vi "TC110.vi"(7 "Function":T3=enum."Read command", 8 "Error in":errorcluster, 10 "Settings in":T2) -> (0 "Error out":errorcluster, 1 "Status_string":string, 2 "Settings out":T2, 3 "output cluster":T1)   [LabVIEW 2018]
uses:
  Ctl/Function_of_TC110.ctl
  PublicSubVI/Ctl/_ctl_RT_TurboSettings.ctl
  Example/RS485_TurboPump/Public/Turbopumps/PV Operating adjustment - Cluster.ctl
  Example/RS485_TurboPump/Pfeiffer Vacuum.lvlib
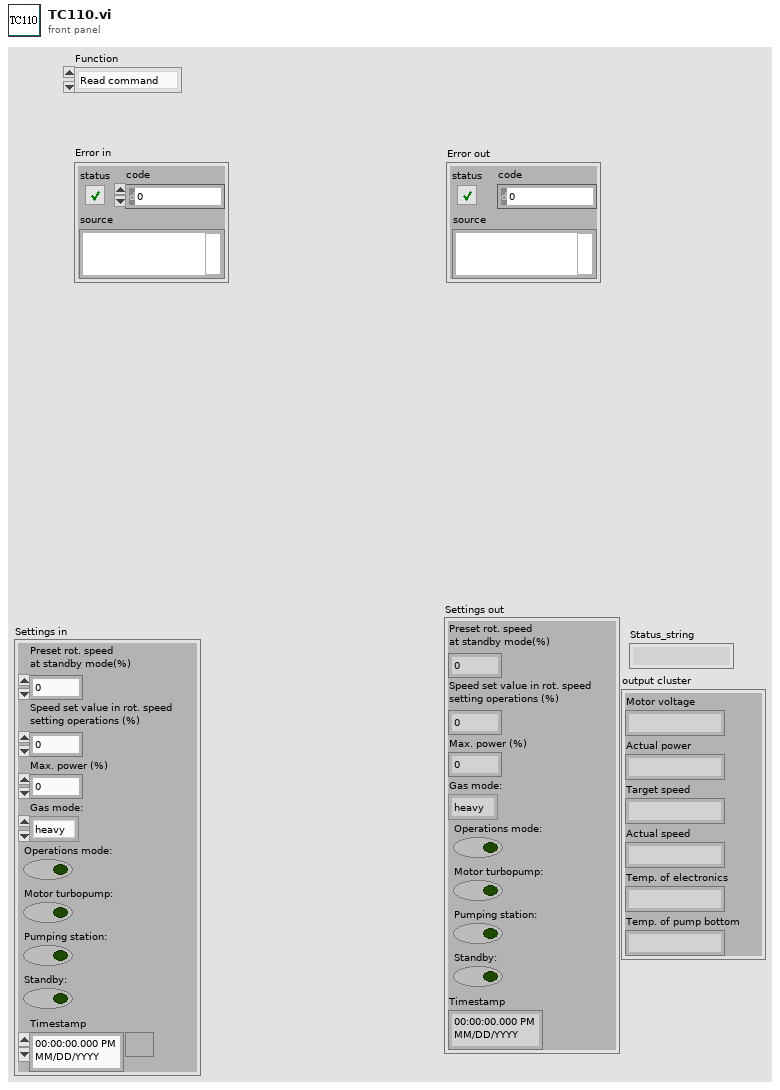
[diagram p1: front panel]
types:
  T1 = cluster{"Motor voltage":string, "Actual power":string, "Target speed":string, "Actual speed":string, "Temp. of electronics":string, "Temp. of pump bottom":string}
  T2 = typedef "_ctl_RT_TurboSettings.ctl" = cluster{"Preset rot. speed \nat standby mode(%)":dbl, "Speed set value in rot. speed \nsetting operations (%)":dbl, "Max. power (%)":dbl, "Gas mode: ":enum16{"heavy", "light", "helium"}, "Operations mode: ":bool, "Motor turbopump: ":bool, "Pumping station: ":bool, "Standby: ":bool, "Timestamp":timestamp}
  T3 = typedef "Function_of_TC110.ctl" = enum16{"Initialisation", "Read status", "Write command", "Read command"}
  T4 = typedef "Pfeiffer Vacuum.lvlib/PV Operating adjustment - Cluster.ctl" = cluster{"Parameter":u16, "Parameter\nread only<->describe":bool, "off<->on":bool, "Rotation speed set value\nin rot. speed setting\noperations [%]":dbl, "Preset rotation Speed\nat Standby mode (%)":dbl, "maximum power\nsetpoint [%]":i32, "Gas mode":u16}
  T5 = enum16{"temperature inverter [°C] (324)", "temperature electronic [°C] (326)", "temperature pump bottom [°C] (330)", "temperature bearing [°C] (342)", "temperature motor [°C] (346)", "temperature rotor [°C] (384)"}
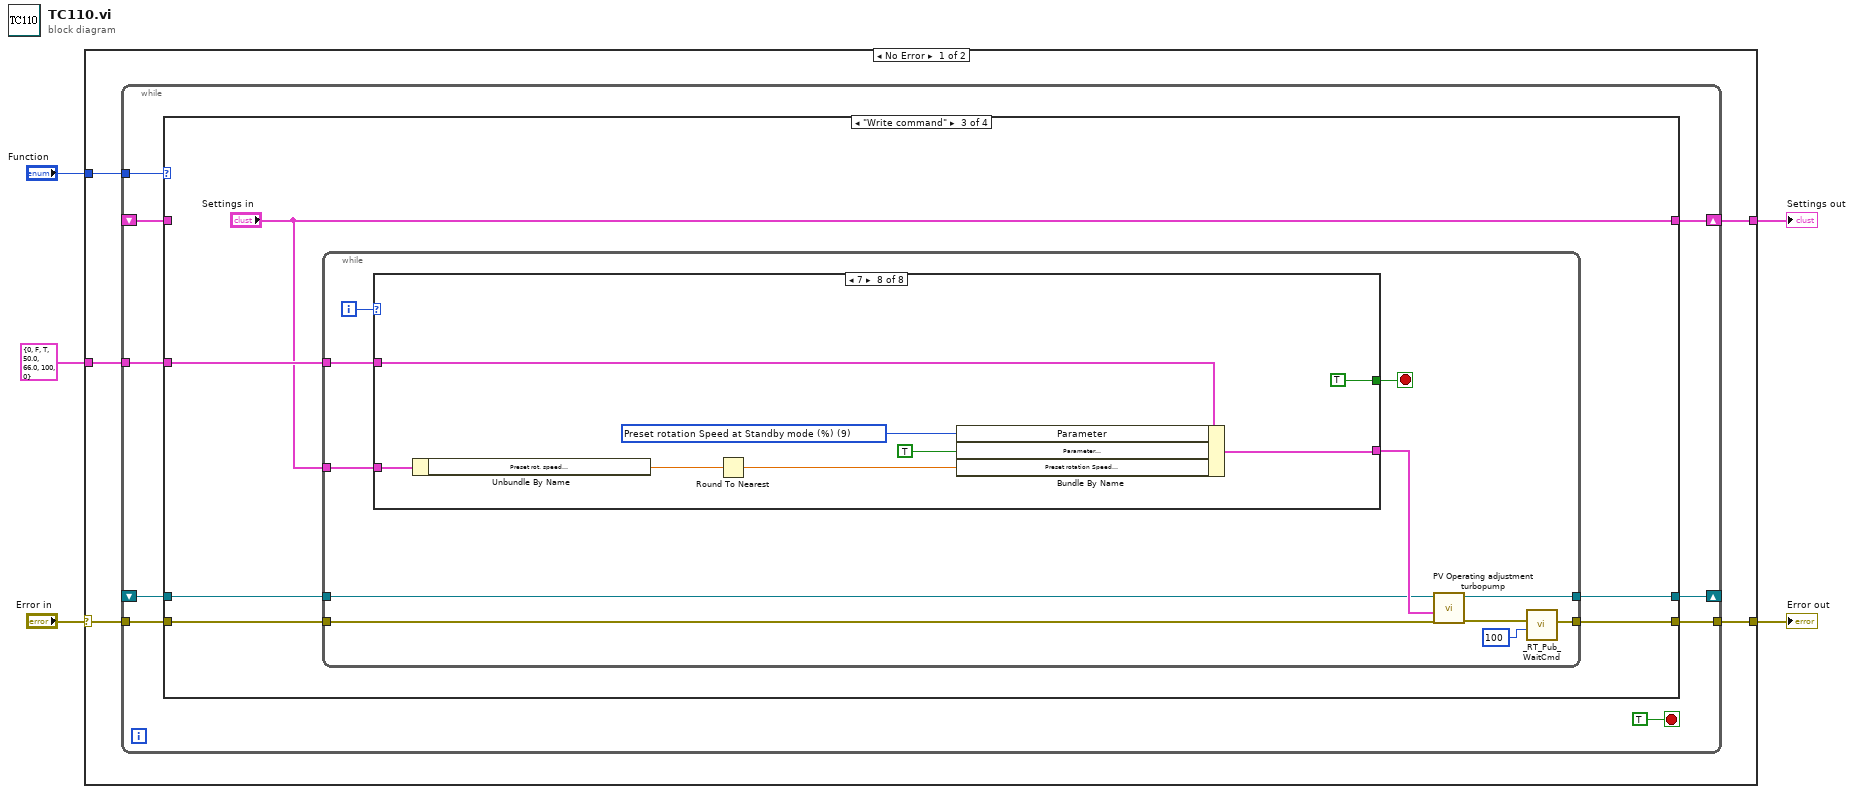
[diagram p0: block diagram]
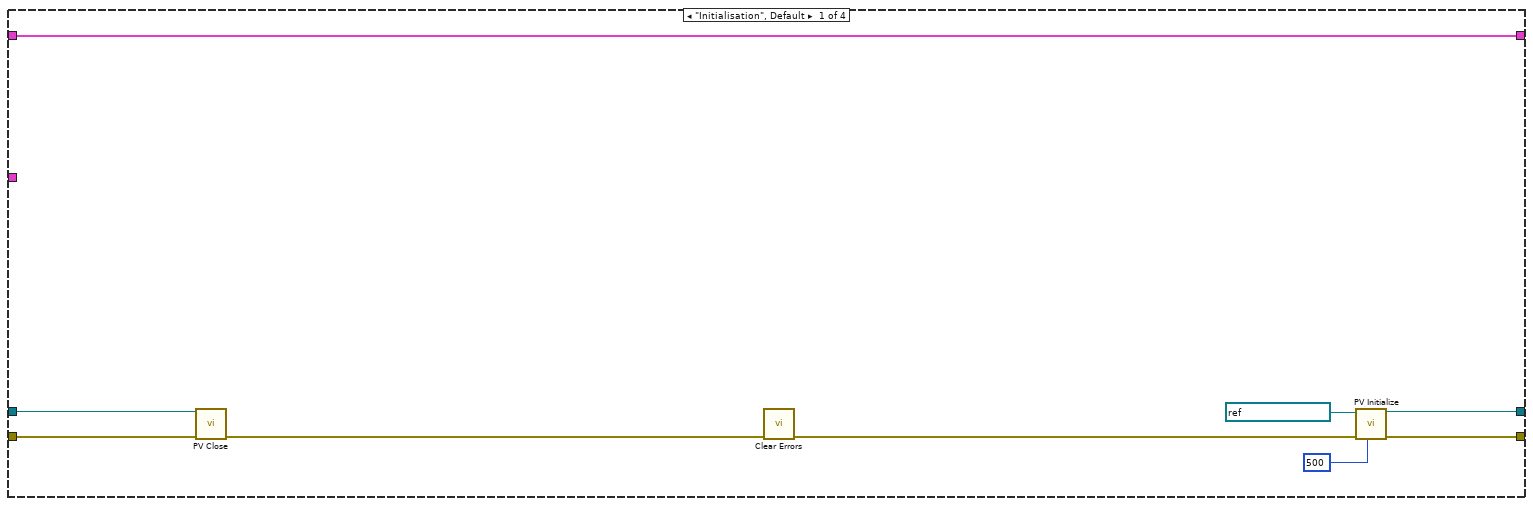
[diagram p2: hidden frame]
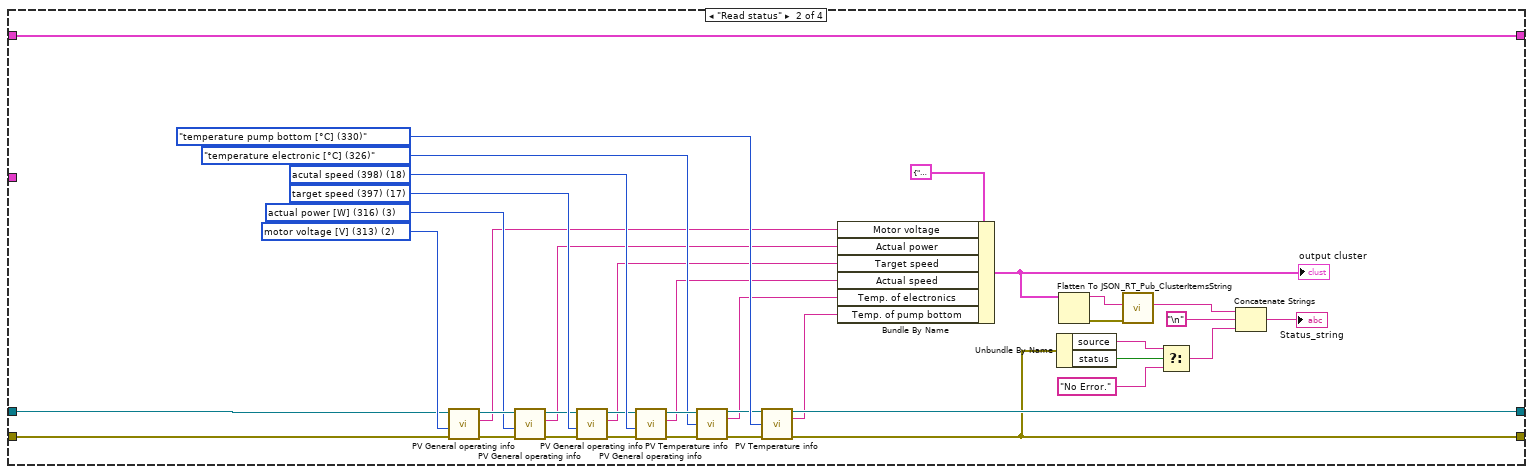
[diagram p3: hidden frame]
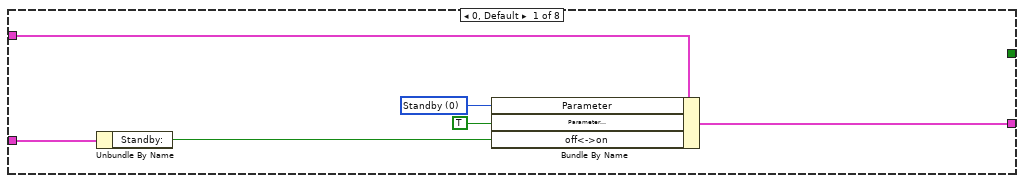
[diagram p4: hidden frame]
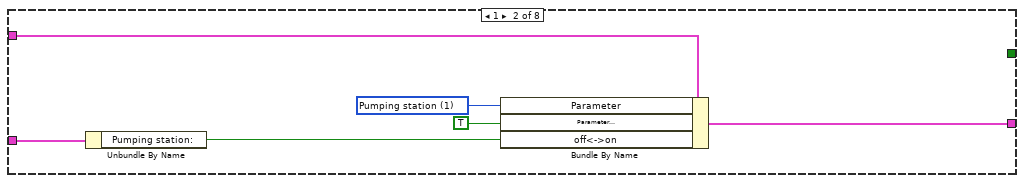
[diagram p5: hidden frame]
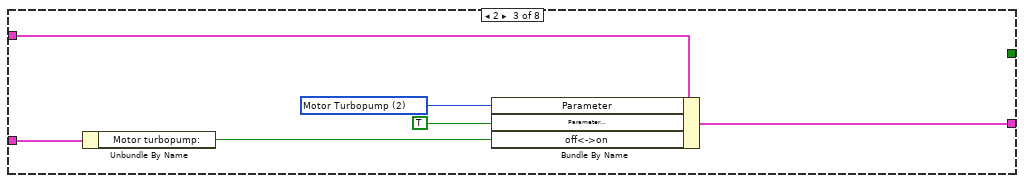
[diagram p6: hidden frame]
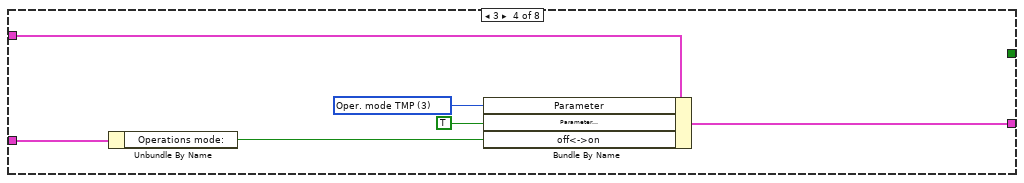
[diagram p7: hidden frame]
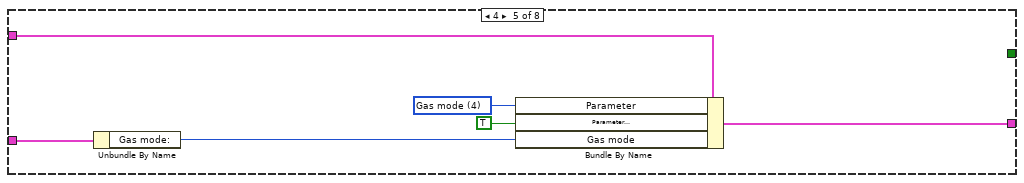
[diagram p8: hidden frame]
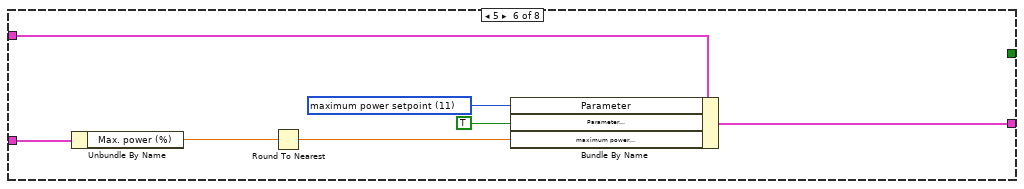
[diagram p9: hidden frame]
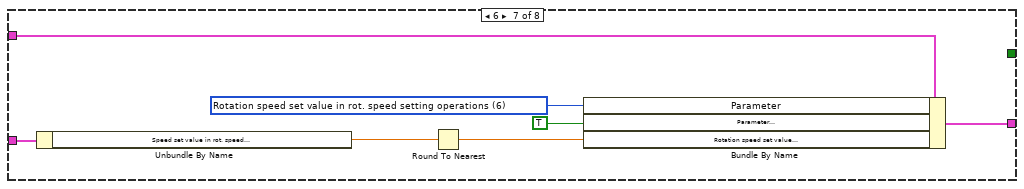
[diagram p10: hidden frame]
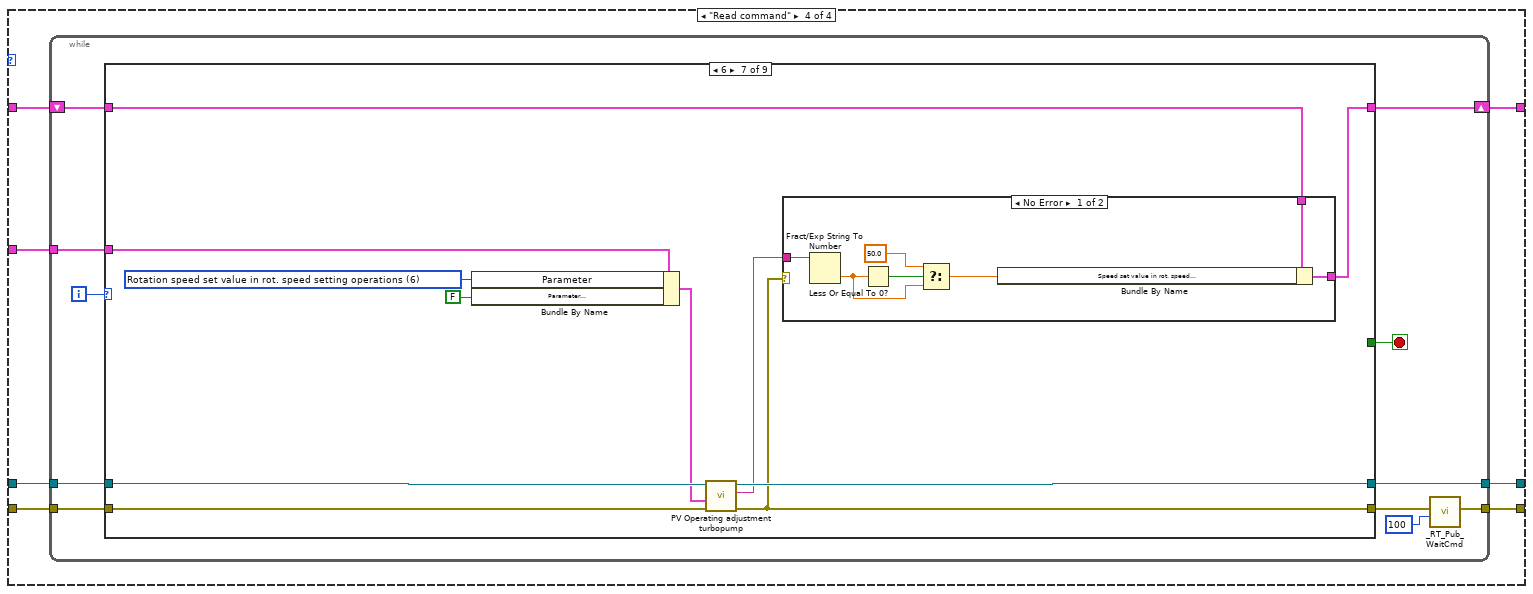
[diagram p11: hidden frame]
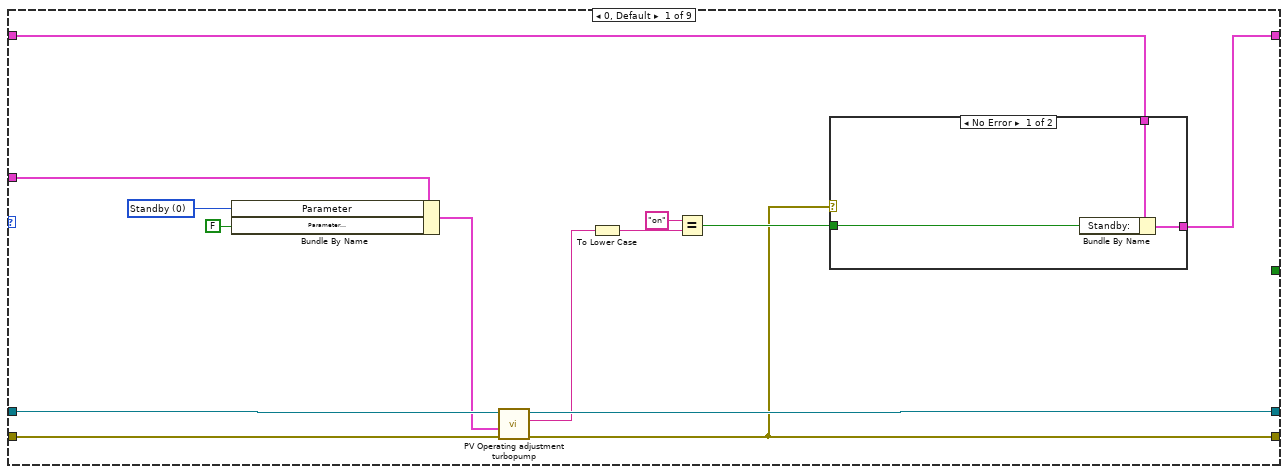
[diagram p12: hidden frame]
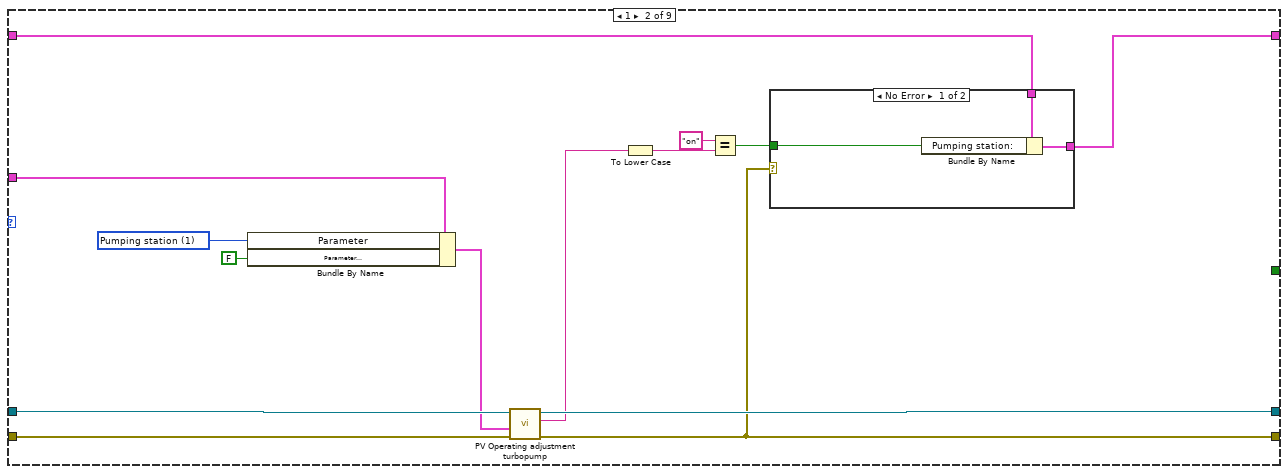
[diagram p14: hidden frame]
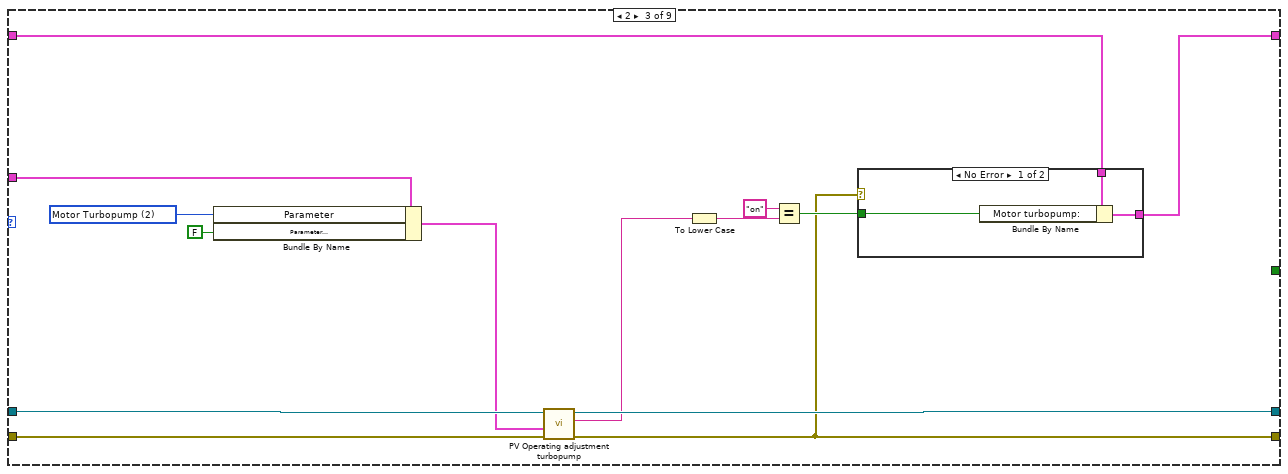
[diagram p16: hidden frame]
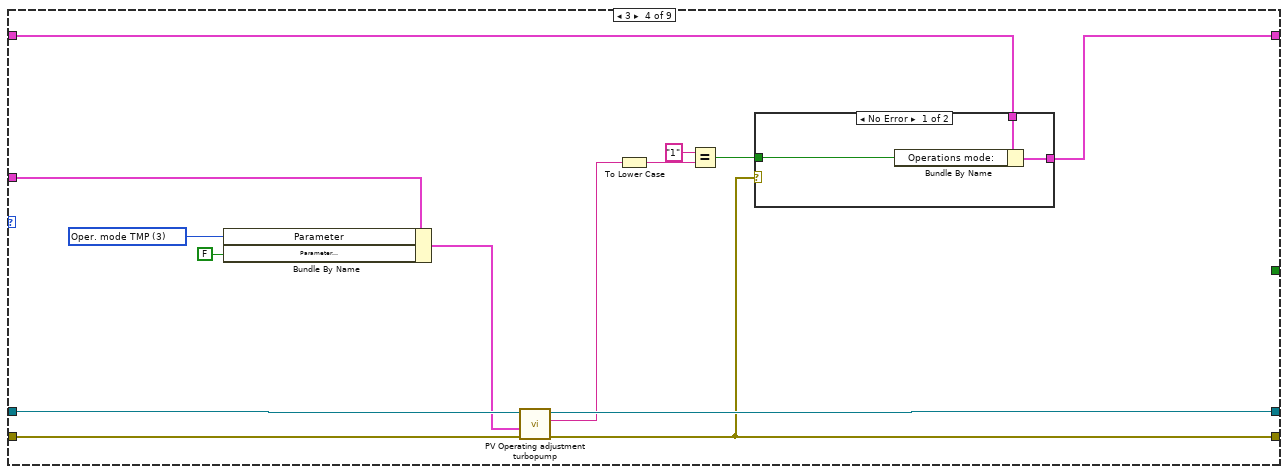
[diagram p18: hidden frame]
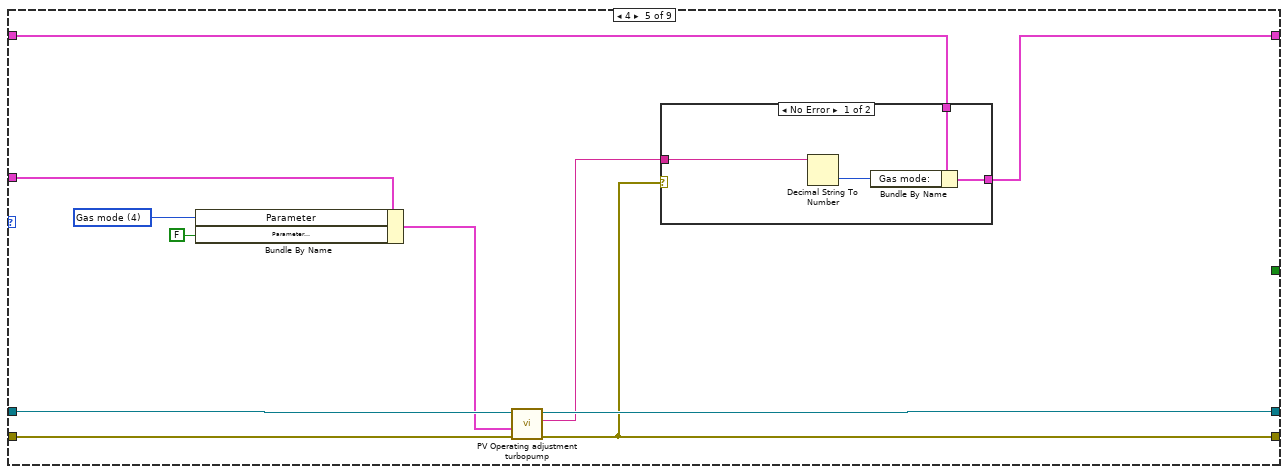
[diagram p20: hidden frame]
diagram:
  n1 = case shown="No Error" "Error in" {
    selector: "Error in" -> [w6 w311]
    tunnel: [w10 w311] -> w5
    tunnel: [w9 _] -> w4
    tunnel: T4 {"Parameter"=0, "Parameter\nread only<->describe"=FALSE, "off<->on"=TRUE, "Rotation speed set value\nin rot. speed setting\noperations [%]"=50.0, "Preset rotation Speed\nat Standby mode (%)"=66.0, "maximum power\nsetpoint [%]"=100, "Gas mode"=0} ("Operating adjustment - Cluster") -> [w8 _]
    tunnel: "Function" -> [w7 _]
    frame No Error {
      n2 = while {
        tunnel: w8 -> [w16]
        tunnel: w7 -> [w14]
        shift-right: [w18] -> w9
        shift-left: _ -> [w15]
        tunnel: w6 -> [w17]
        tunnel: [w19] -> w10
        shift-right: [w13] -> _
        shift-left: _ -> [w11]
        stop <- TRUE stop-if-true
        n3 = case shown="\"Write command\"" w14 {
          tunnel: w17 -> [w24 w30 w70 w140]
          tunnel: [w27 w46 w68 w137] -> w13
          tunnel: w11 -> [w25 w31 w71 w141]
          tunnel: [w26 w39 w69 w138] -> w19
          tunnel: w15 -> [w20 w29 _ w139]
          tunnel: w16 -> [_ _ w72 w142]
          tunnel: [w20 w29 "Settings in" w136] -> w18
          frame "Initialisation", Default {
            n4 = call "PV Close.vi"("VISA session"=w25, "error in (no error)"=w24) -> ("error out"=w23:errorcluster)  [unwired: 13 in]
            n5 = call <vilib>:"Clear Errors.vi"("error in (no error)"=w23) -> ("error out"=w22:errorcluster)  [unwired: 5 in, 1 out]
            n6 = call "PV Initialize.vi"("Timeout Value"=u32 500, "error in (no error)"=w22, "VISA session in"=refnum<visa-resource-name> "ASRL3::INSTR") -> ("error out"=w26:errorcluster, "VISA session out"=w27:refnum<visa-resource-name>)  [unwired: 7 in]
          }
          frame "Read status" {
            w62 = u16 18 items=["nominal speed [Hz] (default) (315)", "intermediate circut current [A] (310)", "motor voltage [V] (313)", "actual power [W] (316)", "operating hours pump [h] (311)", "operating hours drive [h] (314)", "pump cycles (read only) (319)", "status oil sensor (read only) (301)", "speed switchpoint attained (read only) (302)", "overtemperature drive (read only) (304)", "overtemperature pump (read only) (305)", "target speed attained (read only) (306)", "pump accelerates (read only) (307) ", "controlled by remote (300)", "motor phase current [A] (317)", "acceleration / deceleration [rm/s] (336)", "hardware version controller (354)", "target speed (397)", "acutal speed (398)", "nominal speed (399)", "software version control unit (read only) (352)"] ("Parameter")
            w63 = u16 17 items=["nominal speed [Hz] (default) (315)", "intermediate circut current [A] (310)", "motor voltage [V] (313)", "actual power [W] (316)", "operating hours pump [h] (311)", "operating hours drive [h] (314)", "pump cycles (read only) (319)", "status oil sensor (read only) (301)", "speed switchpoint attained (read only) (302)", "overtemperature drive (read only) (304)", "overtemperature pump (read only) (305)", "target speed attained (read only) (306)", "pump accelerates (read only) (307) ", "controlled by remote (300)", "motor phase current [A] (317)", "acceleration / deceleration [rm/s] (336)", "hardware version controller (354)", "target speed (397)", "acutal speed (398)", "nominal speed (399)", "software version control unit (read only) (352)"] ("Parameter")
            w64 = u16 3 items=["nominal speed [Hz] (default) (315)", "intermediate circut current [A] (310)", "motor voltage [V] (313)", "actual power [W] (316)", "operating hours pump [h] (311)", "operating hours drive [h] (314)", "pump cycles (read only) (319)", "status oil sensor (read only) (301)", "speed switchpoint attained (read only) (302)", "overtemperature drive (read only) (304)", "overtemperature pump (read only) (305)", "target speed attained (read only) (306)", "pump accelerates (read only) (307) ", "controlled by remote (300)", "motor phase current [A] (317)", "acceleration / deceleration [rm/s] (336)", "hardware version controller (354)", "target speed (397)", "acutal speed (398)", "nominal speed (399)", "software version control unit (read only) (352)"] ("Parameter")
            w66 = u16 2 items=["nominal speed [Hz] (default) (315)", "intermediate circut current [A] (310)", "motor voltage [V] (313)", "actual power [W] (316)", "operating hours pump [h] (311)", "operating hours drive [h] (314)", "pump cycles (read only) (319)", "status oil sensor (read only) (301)", "speed switchpoint attained (read only) (302)", "overtemperature drive (read only) (304)", "overtemperature pump (read only) (305)", "target speed attained (read only) (306)", "pump accelerates (read only) (307) ", "controlled by remote (300)", "motor phase current [A] (317)", "acceleration / deceleration [rm/s] (336)", "hardware version controller (354)", "target speed (397)", "acutal speed (398)", "nominal speed (399)", "software version control unit (read only) (352)"] ("Parameter")
            n7 = call "PV General operating info.vi"("error in (no error)"=w30, "Parameter"=w66, "VISA session"=w31) -> ("error out"=w59:errorcluster, "response (data)"=w49:string, "dup VISA session"=w65:refnum<visa-resource-name>)  [unwired: 6 in]
            n8 = call "PV General operating info.vi"("error in (no error)"=w59, "Parameter"=w64, "VISA session"=w65) -> ("error out"=w58:errorcluster, "response (data)"=w43:string, "dup VISA session"=w61:refnum<visa-resource-name>)  [unwired: 6 in]
            n9 = call "PV General operating info.vi"("error in (no error)"=w58, "Parameter"=w63, "VISA session"=w61) -> ("error out"=w57:errorcluster, "response (data)"=w44:string, "dup VISA session"=w60:refnum<visa-resource-name>)  [unwired: 6 in]
            n10 = call "PV General operating info.vi"("error in (no error)"=w57, "Parameter"=w62, "VISA session"=w60) -> ("error out"=w53:errorcluster, "response (data)"=w48:string, "dup VISA session"=w56:refnum<visa-resource-name>)  [unwired: 6 in]
            n11 = call "PV Temperature info.vi"("VISA session"=w56, "Parameter"=T5."temperature electronic [°C] (326)", "error in (no error)"=w53) -> ("dup VISA session"=w52:refnum<visa-resource-name>, "response (data)"=w47:string, "error out"=w51:errorcluster)  [unwired: 10 in]
            n12 = call "PV Temperature info.vi"("VISA session"=w52, "Parameter"=T5."temperature pump bottom [°C] (330)", "error in (no error)"=w51) -> ("dup VISA session"=w46:refnum<visa-resource-name>, "response (data)"=w45:string, "error out"=w39:errorcluster)  [unwired: 10 in]
            n13 = Bundle By Name(cluster=T1 {"Motor voltage"="", "Actual power"="", "Target speed"="", "Actual speed"="", "Temp. of electronics"="", "Temp. of pump bottom"=""}, "Motor voltage"=w49, "Actual power"=w43, "Target speed"=w44, "Actual speed"=w48, "Temp. of electronics"=w47, "Temp. of pump bottom"=w45) -> (w42:T1)
            "output cluster" <- w42
            n14 = Unbundle By Name(w39) -> ("source"=w37:string, "status"=w38:bool)
            n15 = Flatten To JSON(anything=w42) -> (JSON string=w41:string, 11:w40:errorcluster)  [unwired: 2 in]
            n16 = call "_RT_Pub_ClusterItemsString.vi"("error in (no error)"=w40, "JSON string"=w41) -> ("result string"=w35:string)  [unwired: 8 in, 1 out]
            n17 = Select(t=w37, s=w38, f="No Error.") -> (s? t:f=w33:string)
            n18 = Concatenate Strings(w35, "\n" ("string"), w33) -> (→"Status_string":string)
          }
          frame "Write command" {
            n19 = while {
              tunnel: "Settings in" -> [w83]
              tunnel: w71 -> [w76]
              tunnel: w70 -> [w75]
              tunnel: [w79] -> w69
              tunnel: w72 -> [w82]
              tunnel: [w73] -> w68
              i -> [w81]
              stop <- w80 stop-if-true
              n20 = case shown="7" w81 {
                tunnel: w83 -> [w87 w93 w99 w105 w111 w118 w125 w133]
                tunnel: w82 -> [w89 w95 w101 w107 w113 w120 w127 w135]
                tunnel: [_ _ _ _ _ _ _ TRUE] -> w80
                tunnel: [w84 w90 w96 w102 w108 w114 w121 w128] -> w77
                frame 0, Default {
                  w85 = u16 0 items=[" Standby", " Pumping station", " Motor Turbopump", " Oper. mode TMP", " Gas mode", " Operating mode drive unit", " Rotation speed set value in rot. speed setting operations", " Set rotation speed TMP [Hz] (read only)", " Actual rotation speed TMP [Hz] (read only)", " Preset rotation Speed at Standby mode (%)", " Max. rotations speed ", " maximum power setpoint"] ("Parameter")
                  n21 = Unbundle By Name(w87) -> ("Standby:"=w86:bool)
                  n22 = Bundle By Name(cluster=w89, "Parameter"=w85, "Parameter\nread only<->describe"=TRUE ("Parameter\nread only<->describe"), "off<->on"=w86) -> (w84:T4)
                }
                frame 1 {
                  w91 = u16 1 items=[" Standby", " Pumping station", " Motor Turbopump", " Oper. mode TMP", " Gas mode", " Operating mode drive unit", " Rotation speed set value in rot. speed setting operations", " Set rotation speed TMP [Hz] (read only)", " Actual rotation speed TMP [Hz] (read only)", " Preset rotation Speed at Standby mode (%)", " Max. rotations speed ", " maximum power setpoint"] ("Parameter")
                  n23 = Unbundle By Name(w93) -> ("Pumping station:"=w92:bool)
                  n24 = Bundle By Name(cluster=w95, "Parameter"=w91, "Parameter\nread only<->describe"=TRUE ("Parameter\nread only<->describe"), "off<->on"=w92) -> (w90:T4)
                }
                frame 2 {
                  w97 = u16 2 items=[" Standby", " Pumping station", " Motor Turbopump", " Oper. mode TMP", " Gas mode", " Operating mode drive unit", " Rotation speed set value in rot. speed setting operations", " Set rotation speed TMP [Hz] (read only)", " Actual rotation speed TMP [Hz] (read only)", " Preset rotation Speed at Standby mode (%)", " Max. rotations speed ", " maximum power setpoint"] ("Parameter")
                  n25 = Unbundle By Name(w99) -> ("Motor turbopump:"=w98:bool)
                  n26 = Bundle By Name(cluster=w101, "Parameter"=w97, "Parameter\nread only<->describe"=TRUE ("Parameter\nread only<->describe"), "off<->on"=w98) -> (w96:T4)
                }
                frame 3 {
                  w103 = u16 3 items=[" Standby", " Pumping station", " Motor Turbopump", " Oper. mode TMP", " Gas mode", " Operating mode drive unit", " Rotation speed set value in rot. speed setting operations", " Set rotation speed TMP [Hz] (read only)", " Actual rotation speed TMP [Hz] (read only)", " Preset rotation Speed at Standby mode (%)", " Max. rotations speed ", " maximum power setpoint"] ("Parameter")
                  n27 = Unbundle By Name(w105) -> ("Operations mode:"=w104:bool)
                  n28 = Bundle By Name(cluster=w107, "Parameter"=w103, "Parameter\nread only<->describe"=TRUE ("Parameter\nread only<->describe"), "off<->on"=w104) -> (w102:T4)
                }
                frame 4 {
                  w109 = u16 4 items=[" Standby", " Pumping station", " Motor Turbopump", " Oper. mode TMP", " Gas mode", " Operating mode drive unit", " Rotation speed set value in rot. speed setting operations", " Set rotation speed TMP [Hz] (read only)", " Actual rotation speed TMP [Hz] (read only)", " Preset rotation Speed at Standby mode (%)", " Max. rotations speed ", " maximum power setpoint"] ("Parameter")
                  n29 = Unbundle By Name(w111) -> ("Gas mode:"=w110:enum16{"heavy", "light", "helium"})
                  n30 = Bundle By Name(cluster=w113, "Parameter"=w109, "Parameter\nread only<->describe"=TRUE ("Parameter\nread only<->describe"), "Gas mode"=w110) -> (w108:T4)
                }
                frame 5 {
                  w116 = u16 11 items=[" Standby", " Pumping station", " Motor Turbopump", " Oper. mode TMP", " Gas mode", " Operating mode drive unit", " Rotation speed set value in rot. speed setting operations", " Set rotation speed TMP [Hz] (read only)", " Actual rotation speed TMP [Hz] (read only)", " Preset rotation Speed at Standby mode (%)", " Max. rotations speed ", " maximum power setpoint"] ("Parameter")
                  n31 = Unbundle By Name(w118) -> ("Max. power (%)"=w117:dbl)
                  n32 = Round To Nearest(number=w117) -> (nearest integer value=w115:dbl)
                  n33 = Bundle By Name(cluster=w120, "Parameter"=w116, "Parameter\nread only<->describe"=TRUE ("Parameter\nread only<->describe"), "maximum power\nsetpoint [%]"=w115) -> (w114:T4)
                }
                frame 6 {
                  w123 = u16 6 items=[" Standby", " Pumping station", " Motor Turbopump", " Oper. mode TMP", " Gas mode", " Operating mode drive unit", " Rotation speed set value in rot. speed setting operations", " Set rotation speed TMP [Hz] (read only)", " Actual rotation speed TMP [Hz] (read only)", " Preset rotation Speed at Standby mode (%)", " Max. rotations speed ", " maximum power setpoint"] ("Parameter")
                  n34 = Unbundle By Name(w125) -> ("Speed set value in rot. speed \nsetting operations (%)"=w124:dbl)
                  n35 = Round To Nearest(number=w124) -> (nearest integer value=w122:dbl)
                  n36 = Bundle By Name(cluster=w127, "Parameter"=w123, "Parameter\nread only<->describe"=TRUE ("Parameter\nread only<->describe"), "Rotation speed set value\nin rot. speed setting\noperations [%]"=w122) -> (w121:T4)
                }
                frame 7 {
                  w131 = u16 9 items=[" Standby", " Pumping station", " Motor Turbopump", " Oper. mode TMP", " Gas mode", " Operating mode drive unit", " Rotation speed set value in rot. speed setting operations", " Set rotation speed TMP [Hz] (read only)", " Actual rotation speed TMP [Hz] (read only)", " Preset rotation Speed at Standby mode (%)", " Max. rotations speed ", " maximum power setpoint"] ("Parameter")
                  n37 = Unbundle By Name(w133) -> ("Preset rot. speed \nat standby mode(%)"=w132:dbl)
                  n38 = Round To Nearest(number=w132) -> (nearest integer value=w130:dbl)
                  n39 = Bundle By Name(cluster=w135, "Parameter"=w131, "Parameter\nread only<->describe"=TRUE ("Parameter\nread only<->describe"), "Preset rotation Speed\nat Standby mode (%)"=w130) -> (w128:T4)
                }
              }
              n40 = call "PV Operating adjustment turbopump.vi"("error in (no error)"=w75, "Operating adjustment - Cluster"=w77, "VISA session"=w76) -> ("error out"=w74:errorcluster, "dup VISA session"=w73:refnum<visa-resource-name>)  [unwired: 6 in, 1 out]
              n41 = call "_RT_Pub_WaitCmd.vi"("milliseconds to wait"=u32 100, "error in (no error)"=w74) -> ("error out"=w79:errorcluster)  [unwired: 9 in]
            }
          }
          frame "Read command" {
            n42 = while {
              tunnel: w141 -> [w150]
              tunnel: w140 -> [w149]
              tunnel: [w151] -> w137
              tunnel: [w143] -> w138
              shift-right: [w147] -> w136
              shift-left: w139 -> [w146]
              tunnel: w142 -> [w153]
              i -> [w152]
              stop <- w148 stop-if-true
              n43 = case shown="6" w152 {
                tunnel: w153 -> [w158 w185 w203 w221 w236 w252 w271 w290 _]
                tunnel: [w166 w183 w201 w219 w234 w250 w269 w288 w302] -> w151
                tunnel: w150 -> [w165 w182 w200 w218 w233 w249 w268 w287 w302]
                tunnel: [w155 w172 w192 w211 w228 w244 w264 w283 w301] -> w144
                tunnel: w149 -> [w163 w180 w198 w216 w231 w248 w266 w286 w301]
                tunnel: [_ _ _ _ _ _ _ _ TRUE] -> w148
                tunnel: [w156 w175 w190 w208 w226 w242 w261 w280 w304] -> w147
                tunnel: w146 -> [w154 w173 w191 w209 w227 w243 w262 w281 w306]
                frame 0, Default {
                  w162 = u16 0 items=[" Standby", " Pumping station", " Motor Turbopump", " Oper. mode TMP", " Gas mode", " Operating mode drive unit", " Rotation speed set value in rot. speed setting operations", " Set rotation speed TMP [Hz] (read only)", " Actual rotation speed TMP [Hz] (read only)", " Preset rotation Speed at Standby mode (%)", " Max. rotations speed ", " maximum power setpoint"] ("Parameter")
                  n44 = Bundle By Name(cluster=w158, "Parameter"=w162, "Parameter\nread only<->describe"=FALSE ("Parameter\nread only<->describe")) -> (w164:T4)
                  n45 = call "PV Operating adjustment turbopump.vi"("error in (no error)"=w163, "Operating adjustment - Cluster"=w164, "VISA session"=w165) -> ("error out"=w155:errorcluster, "response (data)"=w159:string, "dup VISA session"=w166:refnum<visa-resource-name>)  [unwired: 6 in]
                  n46 = To Lower Case(string=w159) -> (all lower case string=w160:string)
                  n47 = Equal?(x="on", y=w160) -> (x = y?=w157:bool)
                  n48 = case shown="No Error" w155 {
                    tunnel: w157 -> [w170 _]
                    tunnel: [w169 w171] -> w156
                    tunnel: w154 -> [w168 w171]
                    frame No Error {
                      n49 = Bundle By Name(cluster=w168, "Standby:"=w170) -> (w169:T2)
                    }
                    frame Error {
                    }
                  }
                }
                frame 1 {
                  w179 = u16 1 items=[" Standby", " Pumping station", " Motor Turbopump", " Oper. mode TMP", " Gas mode", " Operating mode drive unit", " Rotation speed set value in rot. speed setting operations", " Set rotation speed TMP [Hz] (read only)", " Actual rotation speed TMP [Hz] (read only)", " Preset rotation Speed at Standby mode (%)", " Max. rotations speed ", " maximum power setpoint"] ("Parameter")
                  n50 = Bundle By Name(cluster=w185, "Parameter"=w179, "Parameter\nread only<->describe"=FALSE ("Parameter\nread only<->describe")) -> (w181:T4)
                  n51 = call "PV Operating adjustment turbopump.vi"("error in (no error)"=w180, "Operating adjustment - Cluster"=w181, "VISA session"=w182) -> ("error out"=w172:errorcluster, "response (data)"=w174:string, "dup VISA session"=w183:refnum<visa-resource-name>)  [unwired: 6 in]
                  n52 = To Lower Case(string=w174) -> (all lower case string=w177:string)
                  n53 = Equal?(x="on", y=w177) -> (x = y?=w176:bool)
                  n54 = case shown="No Error" w172 {
                    tunnel: w176 -> [w188 _]
                    tunnel: [w187 w189] -> w175
                    tunnel: w173 -> [w186 w189]
                    frame No Error {
                      n55 = Bundle By Name(cluster=w186, "Pumping station:"=w188) -> (w187:T2)
                    }
                    frame Error {
                    }
                  }
                }
                frame 2 {
                  w197 = u16 2 items=[" Standby", " Pumping station", " Motor Turbopump", " Oper. mode TMP", " Gas mode", " Operating mode drive unit", " Rotation speed set value in rot. speed setting operations", " Set rotation speed TMP [Hz] (read only)", " Actual rotation speed TMP [Hz] (read only)", " Preset rotation Speed at Standby mode (%)", " Max. rotations speed ", " maximum power setpoint"] ("Parameter")
                  n56 = Bundle By Name(cluster=w203, "Parameter"=w197, "Parameter\nread only<->describe"=FALSE ("Parameter\nread only<->describe")) -> (w199:T4)
                  n57 = call "PV Operating adjustment turbopump.vi"("error in (no error)"=w198, "Operating adjustment - Cluster"=w199, "VISA session"=w200) -> ("error out"=w192:errorcluster, "response (data)"=w193:string, "dup VISA session"=w201:refnum<visa-resource-name>)  [unwired: 6 in]
                  n58 = To Lower Case(string=w193) -> (all lower case string=w195:string)
                  n59 = Equal?(x="on", y=w195) -> (x = y?=w194:bool)
                  n60 = case shown="No Error" w192 {
                    tunnel: w194 -> [w206 _]
                    tunnel: [w205 w207] -> w190
                    tunnel: w191 -> [w204 w207]
                    frame No Error {
                      n61 = Bundle By Name(cluster=w204, "Motor turbopump:"=w206) -> (w205:T2)
                    }
                    frame Error {
                    }
                  }
                }
                frame 3 {
                  w215 = u16 3 items=[" Standby", " Pumping station", " Motor Turbopump", " Oper. mode TMP", " Gas mode", " Operating mode drive unit", " Rotation speed set value in rot. speed setting operations", " Set rotation speed TMP [Hz] (read only)", " Actual rotation speed TMP [Hz] (read only)", " Preset rotation Speed at Standby mode (%)", " Max. rotations speed ", " maximum power setpoint"] ("Parameter")
                  n62 = Bundle By Name(cluster=w221, "Parameter"=w215, "Parameter\nread only<->describe"=FALSE ("Parameter\nread only<->describe")) -> (w217:T4)
                  n63 = call "PV Operating adjustment turbopump.vi"("error in (no error)"=w216, "Operating adjustment - Cluster"=w217, "VISA session"=w218) -> ("error out"=w211:errorcluster, "response (data)"=w212:string, "dup VISA session"=w219:refnum<visa-resource-name>)  [unwired: 6 in]
                  n64 = To Lower Case(string=w212) -> (all lower case string=w214:string)
                  n65 = Equal?(x="1", y=w214) -> (x = y?=w213:bool)
                  n66 = case shown="No Error" w211 {
                    tunnel: w213 -> [w224 _]
                    tunnel: [w223 w225] -> w208
                    tunnel: w209 -> [w222 w225]
                    frame No Error {
                      n67 = Bundle By Name(cluster=w222, "Operations mode:"=w224) -> (w223:T2)
                    }
                    frame Error {
                    }
                  }
                }
                frame 4 {
                  w230 = u16 4 items=[" Standby", " Pumping station", " Motor Turbopump", " Oper. mode TMP", " Gas mode", " Operating mode drive unit", " Rotation speed set value in rot. speed setting operations", " Set rotation speed TMP [Hz] (read only)", " Actual rotation speed TMP [Hz] (read only)", " Preset rotation Speed at Standby mode (%)", " Max. rotations speed ", " maximum power setpoint"] ("Parameter")
                  n68 = Bundle By Name(cluster=w236, "Parameter"=w230, "Parameter\nread only<->describe"=FALSE ("Parameter\nread only<->describe")) -> (w232:T4)
                  n69 = call "PV Operating adjustment turbopump.vi"("error in (no error)"=w231, "Operating adjustment - Cluster"=w232, "VISA session"=w233) -> ("error out"=w228:errorcluster, "response (data)"=w229:string, "dup VISA session"=w234:refnum<visa-resource-name>)  [unwired: 6 in]
                  n70 = case shown="No Error" w228 {
                    tunnel: w229 -> [w240 _]
                    tunnel: w227 -> [w238 w241]
                    tunnel: [w237 w241] -> w226
                    frame No Error {
                      n71 = Decimal String To Number(string=w240) -> (number=w239:i32)  [unwired: 2 in, 1 out]
                      n72 = Bundle By Name(cluster=w238, "Gas mode:"=w239) -> (w237:T2)
                    }
                    frame Error {
                    }
                  }
                }
                frame 5 {
                  w247 = u16 11 items=[" Standby", " Pumping station", " Motor Turbopump", " Oper. mode TMP", " Gas mode", " Operating mode drive unit", " Rotation speed set value in rot. speed setting operations", " Set rotation speed TMP [Hz] (read only)", " Actual rotation speed TMP [Hz] (read only)", " Preset rotation Speed at Standby mode (%)", " Max. rotations speed ", " maximum power setpoint"] ("Parameter")
                  n73 = Bundle By Name(cluster=w252, "Parameter"=w247, "Parameter\nread only<->describe"=FALSE ("Parameter\nread only<->describe")) -> (w246:T4)
                  n74 = call "PV Operating adjustment turbopump.vi"("error in (no error)"=w248, "Operating adjustment - Cluster"=w246, "VISA session"=w249) -> ("error out"=w244:errorcluster, "response (data)"=w245:string, "dup VISA session"=w250:refnum<visa-resource-name>)  [unwired: 6 in]
                  n75 = case shown="No Error" w244 {
                    tunnel: w245 -> [w259 _]
                    tunnel: w243 -> [w258 w260]
                    tunnel: [w257 w260] -> w242
                    frame No Error {
                      n76 = Fract/Exp String To Number(string=w259) -> (number=w254:dbl)  [unwired: 3 in, 1 out]
                      n77 = Less Or Equal To 0?(x=w254) -> (x <= 0?=w256:bool)
                      n78 = Select(t=80.0, s=w256, f=w254) -> (s? t:f=w253:dbl)
                      n79 = Bundle By Name(cluster=w258, "Max. power (%)"=w253) -> (w257:T2)
                    }
                    frame Error {
                    }
                  }
                }
                frame 6 {
                  w265 = u16 6 items=[" Standby", " Pumping station", " Motor Turbopump", " Oper. mode TMP", " Gas mode", " Operating mode drive unit", " Rotation speed set value in rot. speed setting operations", " Set rotation speed TMP [Hz] (read only)", " Actual rotation speed TMP [Hz] (read only)", " Preset rotation Speed at Standby mode (%)", " Max. rotations speed ", " maximum power setpoint"] ("Parameter")
                  n80 = Bundle By Name(cluster=w271, "Parameter"=w265, "Parameter\nread only<->describe"=FALSE ("Parameter\nread only<->describe")) -> (w267:T4)
                  n81 = call "PV Operating adjustment turbopump.vi"("error in (no error)"=w266, "Operating adjustment - Cluster"=w267, "VISA session"=w268) -> ("error out"=w264:errorcluster, "response (data)"=w263:string, "dup VISA session"=w269:refnum<visa-resource-name>)  [unwired: 6 in]
                  n82 = case shown="No Error" w264 {
                    tunnel: w263 -> [w278 _]
                    tunnel: [w277 w279] -> w261
                    tunnel: w262 -> [w276 w279]
                    frame No Error {
                      n83 = Fract/Exp String To Number(string=w278) -> (number=w273:dbl)  [unwired: 3 in, 1 out]
                      n84 = Less Or Equal To 0?(x=w273) -> (x <= 0?=w275:bool)
                      n85 = Select(t=50.0, s=w275, f=w273) -> (s? t:f=w272:dbl)
                      n86 = Bundle By Name(cluster=w276, "Speed set value in rot. speed \nsetting operations (%)"=w272) -> (w277:T2)
                    }
                    frame Error {
                    }
                  }
                }
                frame 7 {
                  w285 = u16 9 items=[" Standby", " Pumping station", " Motor Turbopump", " Oper. mode TMP", " Gas mode", " Operating mode drive unit", " Rotation speed set value in rot. speed setting operations", " Set rotation speed TMP [Hz] (read only)", " Actual rotation speed TMP [Hz] (read only)", " Preset rotation Speed at Standby mode (%)", " Max. rotations speed ", " maximum power setpoint"] ("Parameter")
                  n87 = Bundle By Name(cluster=w290, "Parameter"=w285, "Parameter\nread only<->describe"=FALSE ("Parameter\nread only<->describe")) -> (w284:T4)
                  n88 = call "PV Operating adjustment turbopump.vi"("error in (no error)"=w286, "Operating adjustment - Cluster"=w284, "VISA session"=w287) -> ("error out"=w283:errorcluster, "response (data)"=w282:string, "dup VISA session"=w288:refnum<visa-resource-name>)  [unwired: 6 in]
                  n89 = case shown="No Error" w283 {
                    tunnel: [w297 w300] -> w280
                    tunnel: w282 -> [w296 _]
                    tunnel: w281 -> [w295 w300]
                    frame No Error {
                      n90 = Fract/Exp String To Number(string=w296) -> (number=w292:dbl)  [unwired: 3 in, 1 out]
                      n91 = Less Or Equal To 0?(x=w292) -> (x <= 0?=w294:bool)
                      n92 = Select(t=50.0, s=w294, f=w292) -> (s? t:f=w291:dbl)
                      n93 = Divide(x=w291, y=100.0) -> (x/y=w299:dbl)
                      n94 = Bundle By Name(cluster=w295, "Preset rot. speed \nat standby mode(%)"=w299) -> (w297:T2)
                    }
                    frame Error {
                    }
                  }
                }
                frame 8 {
                  n95 = Unbundle By Name(w306) -> ("Timestamp"=w308:timestamp)
                  n96 = Equal?(x=timestamp(0 s since 1904-01-01) ("y"), y=w308) -> (x = y?=w310:bool)
                  n97 = Get Date/Time In Seconds() -> (seconds since 1Jan1904=w307:timestamp)
                  n98 = Select(t=w307, s=w310, f=w308) -> (s? t:f=w305:timestamp)
                  n99 = Bundle By Name(cluster=w306, "Timestamp"=w305) -> (w304:T2)
                }
              }
              n100 = call "_RT_Pub_WaitCmd.vi"("milliseconds to wait"=u32 100, "error in (no error)"=w144) -> ("error out"=w143:errorcluster)  [unwired: 9 in]
            }
          }
        }
      }
    }
    frame Error {
    }
  }
  "Error out" <- w5
  "Settings out" <- w4
